vi "DAQ.Get Device Info.vi"(8 "error in (no error)":errorcluster, 11 "Instrument.DAQ":refnum<class "Instrument.DAQ.lvclass">) -> (0 "error out":errorcluster, 3 "Instrument.DAQ":refnum<class "Instrument.DAQ.lvclass">)   [LabVIEW 2019, in "Instrument.Lockin.lvlib" / "Instrument.DAQ.lvclass"]
uses:
  Instrument.DAQ.lvclass
  Instrument.DAQ.lvclass/Instrument.DAQ.ctl
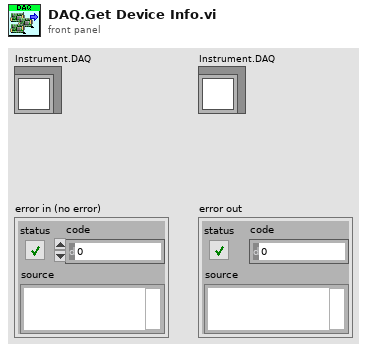
[diagram p1: front panel]
types:
  T1 = typedef "Instrument.Lockin.lvlib/Instrument.DAQ.lvclass/DeviceInfo--Cluster.ctl" = cluster{"DeviceName":string, "DevIsSimulated":bool, "DeviceSerialNumber":string, "ProductType":string, "ProductCategory":i32, "ProductNumber":u32, "ChassisNumber":u32, "SlotNumber":u32, "ChassisName":string, "ChassisSerialNumber":string, "DevTemp":dbl, "SelfCal.LastDate/Time":string, "SelfCal.LastTemp":dbl, "calibration due?":bool}
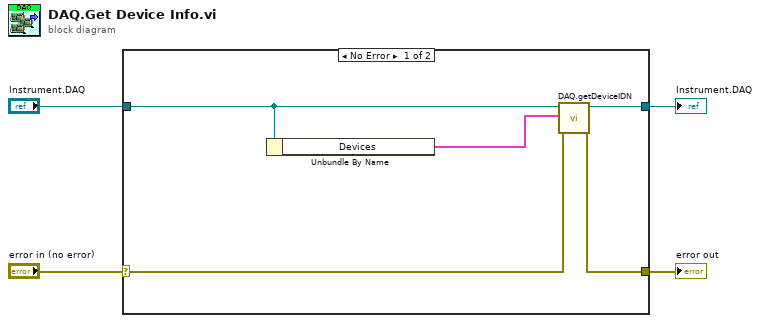
[diagram p0: block diagram]
diagram:
  n1 = case shown="No Error" "error in (no error)" {
    selector: "error in (no error)" -> [w6 w10]
    tunnel: "Instrument.DAQ" -> [w8 w11]
    tunnel: [w9 w11] -> w2
    tunnel: [w7 w10] -> w1
    frame No Error {
      n2 = Unbundle By Name(w8) -> ("Devices"=w5:T1[])
      n3 = call "DAQ.getDeviceIDN.vi"("error in (no error)"=w6, "Devices"=w5, "Instrument.DAQ"=w8) -> ("error out"=w7:errorcluster, "Instrument.DAQ out"=w9:refnum<class "Instrument.DAQ.lvclass">)  [unwired: 7 in]
    }
    frame Error {
    }
  }
  "Instrument.DAQ" <- w2
  "error out" <- w1
